vi "Set message_del.vi"(8 "error in (no error)":errorcluster, 10 "wamplv.lvlib:WampMessage MsgPack.lvclass":refnum<class "WampMessage MsgPack.lvclass">, 11 "WelcomeHandler MsgPack in":refnum<class "WelcomeHandler MsgPack.lvclass">) -> (0 "error out":errorcluster, 3 "WelcomeHandler MsgPack out":refnum<class "WelcomeHandler MsgPack.lvclass">)   [LabVIEW 2020]
uses:
  WelcomeHandler MsgPack.lvclass/WelcomeHandler MsgPack.ctl
  WelcomeHandler MsgPack.lvclass
  C:/local/wamplv/Private/Requests/MessageReceivedHandlers/IReceivedMessageHandler/IReceivedMessageHandler.lvclass
  C:/local/wamplv/Private/Requests/IInternalMessage/IInternalMessage.lvclass
  C:/local/wamplv/Private/Requests/MessageReceivedHandlers/Welcome/IWelcomeHandler/IWelcomeHandler.lvclass
  C:/local/wamplv/Private/Requests/MessageReceivedHandlers/Welcome/WelcomeHandler MsgPack/WelcomeHandler MsgPack.lvclass
  C:/local/wamplv/Private/Requests/MessageReceivedHandlers/IMsgPackMessageHandler/IMsgPackMessageHandler.lvclass
  SerialisedMessages/MsgPackMessage/WampMessage MsgPack.lvclass
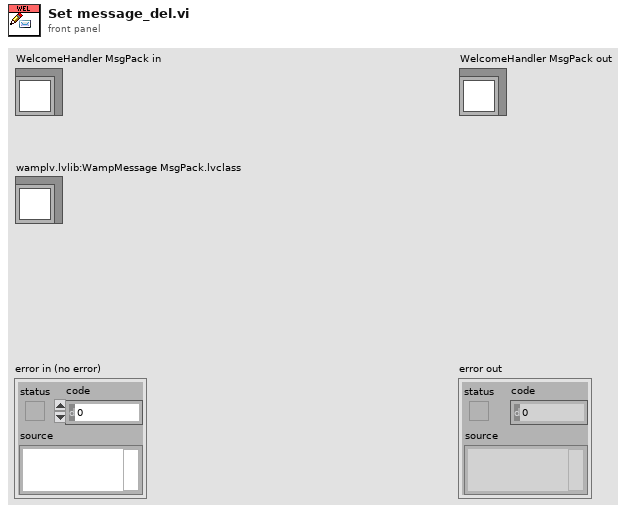
[diagram p1: front panel]
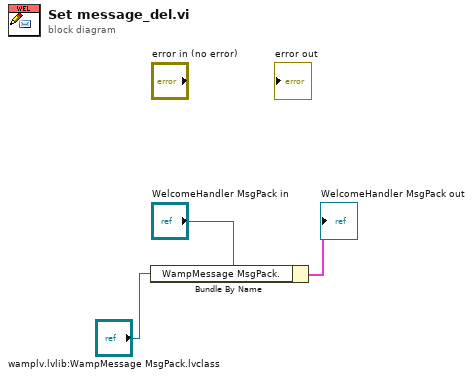
[diagram p0: block diagram]
diagram:
  n1 = Bundle By Name(cluster="WelcomeHandler MsgPack in", "WampMessage MsgPack."="wamplv.lvlib:WampMessage MsgPack.lvclass") -> (→"WelcomeHandler MsgPack out":cluster{})
